vi "RTM - Import from XML.vi"(8 "error in (no error)":errorcluster, 11 "Node Ptr":u64 format="%.0x") -> (0 "error out":errorcluster)   [LabVIEW 2016, in "UDP-Custom-Device System Explorer.lvlib"]
uses:
  UDP-Custom-Device System Explorer.lvlib
  <vilib>/NI VeriStand/Custom Device Tools/Custom Device Utility Library/Custom Device Utility Library.lvlib
panel:
  in  "Tag":string
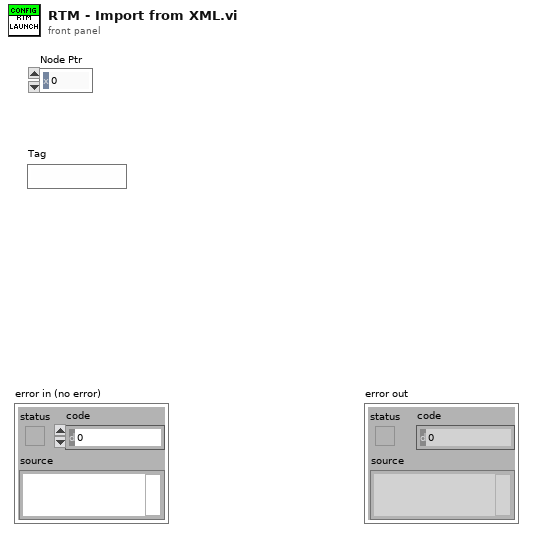
[diagram p1: front panel]
types:
  T1 = typedef "UDP-Custom-Device System Explorer.lvlib/XML - Channel.ctl" = cluster{"Channel Name":string, "Data Type":u16, "Description":string, "Unit":string}
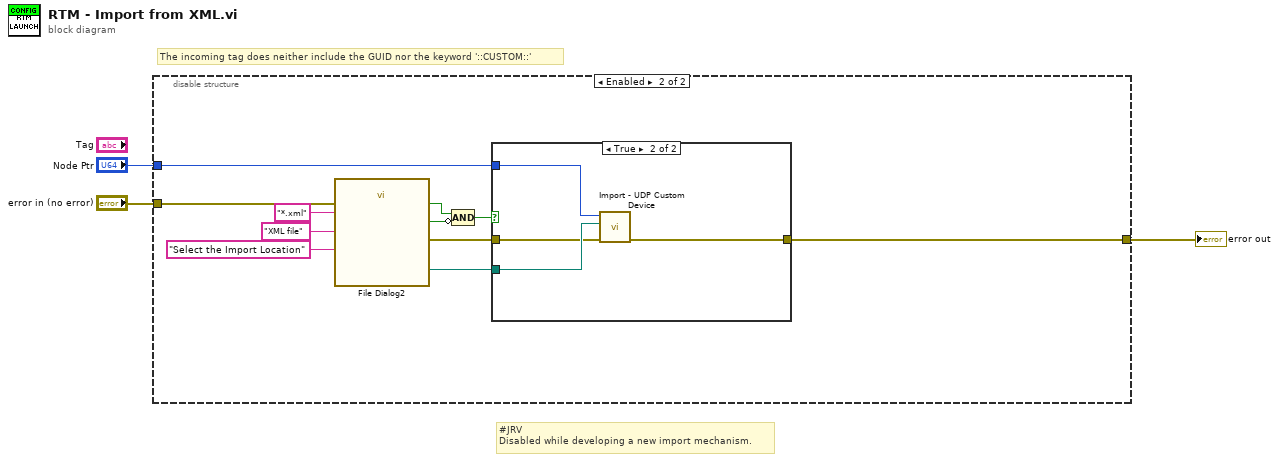
[diagram p0: block diagram]
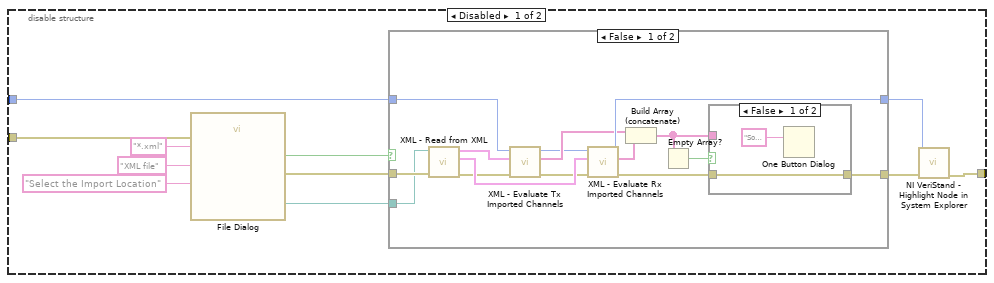
[diagram p2: hidden frame]
diagram:
  # "#JRV\nDisabled while developing a new import mechanism."
  # "The incoming tag does neither include the GUID nor the keyword '::CUSTOM::'"
  n1 = disable-structure shown="Enabled" {
    disable-tunnel: "error in (no error)" -> [w14 w42]
    disable-tunnel: [w6 w39] -> w2
    disable-tunnel: "Node Ptr" -> [w5 w35]
    frame Disabled {
      n2 = call "File Dialog"("prompt"="Select the Import Location", "error in"=w14, "pattern (all files)"="*.xml", "pattern label"="XML file") -> ("selected path"=w8:path, "cancelled"=w10:bool, "error out"=w9:errorcluster)  [unwired: 8 in, 1 out]
      n3 = case shown="False" w10 {
        tunnel: w9 -> [w29 w34]
        tunnel: w8 -> [w28 _]
        tunnel: [w24 w34] -> w7
        tunnel: w5 -> [w20 w33]
        tunnel: [w21 w33] -> w4
        frame False {
          n4 = call "XML - Read from XML.vi"("error in (no error)"=w29, "path to XML document"=w28) -> ("error out"=w18:errorcluster, "Rx Channel Info"=w27:T1[], "Tx Channel Info"=w19:T1[])  [unwired: 7 in]
          n5 = call "XML - Evaluate Tx Imported Channels.vi"("error in (no error)"=w18, "Channel Info Array"=w19, "Node Ptr in"=w20) -> ("error out"=w17:errorcluster, "Invalid Channels"=w16:string[], "Node Ptr out"=w15:u64)  [unwired: 6 in]
          n6 = call "XML - Evaluate Rx Imported Channels.vi"("error in (no error)"=w17, "Channel Info Array"=w27, "Node Ptr in"=w15) -> ("error out"=w25:errorcluster, "Invalid Channels"=w26:string[], "Node Ptr out"=w21:u64)  [unwired: 6 in]
          n7 = Build Array (concatenate)(w16, w26) -> (w22:string[])
          n8 = Empty Array?(array=w22) -> (empty?=w23:bool)
          n9 = case shown="False" w23 {
            tunnel: w25 -> [w31 w32]
            tunnel: [w31 w32] -> w24
            tunnel: w22 -> [_ _]
            frame False {
              n10 = One Button Dialog(message="Some channels were unable to be added because they do not exist in the current system definition.") -> ()  [unwired: 1 in, 1 out]
            }
            frame True {
            }
          }
        }
        frame True {
        }
      }
      n11 = call <vilib>:"NI VeriStand - Highlight Node in System Explorer.vi"("error in (no error)"=w7, "Item Ref in"=w4) -> ("error out"=w6:errorcluster)  [unwired: 8 in, 1 out]
    }
    frame Enabled {
      n12 = call "File Dialog2"("prompt"="Select the Import Location", "error in"=w42, "pattern (all files)"="*.xml", "pattern label"="XML file") -> ("selected path"=w41:path, "exists"=w38:bool, "cancelled"=w37:bool, "error out"=w40:errorcluster)  [unwired: 8 in]
      n13 = Compound Arithmetic op=AND(w38, invert w37) -> (w36:bool)
      n14 = case shown="True" w36 {
        tunnel: w41 -> [_ w50]
        tunnel: w40 -> [w46 w49]
        tunnel: [w46 w48] -> w39
        tunnel: w35 -> [_ w47]
        frame False {
        }
        frame True {
          n15 = call "Import - UDP Custom Device.vi"("error in (no error)"=w49, "Target File"=w50, "Device Item Ref in"=w47) -> ("error out"=w48:errorcluster)  [unwired: 8 in]
        }
      }
    }
  }
  "error out" <- w2
